vi "禹山电导率_获取温度和测量值.vi"(8 "error in (no error)":errorcluster caption="错误输入（无错误）", 11 "MB session in":refnum<class "MB_Master.lvclass">) -> (0 "error out":errorcluster caption="错误输出", 2 "输出值":cluster{"温度测量值":sgl, "电导率":sgl, "错误标志":u16} {"错误标志" items=["NO Error"=0, "量程切换错误标识"=255]}, 3 "MB session out":refnum<class "MB_Master.lvclass">)   [LabVIEW 2016, in "斯坦道多参数.lvlib"]
uses:
  <vilib>/Plasmionique/MB Master/MB_Master/MB_Master.lvclass
  <vilib>/Plasmionique/MB Master/MB Master.lvlib
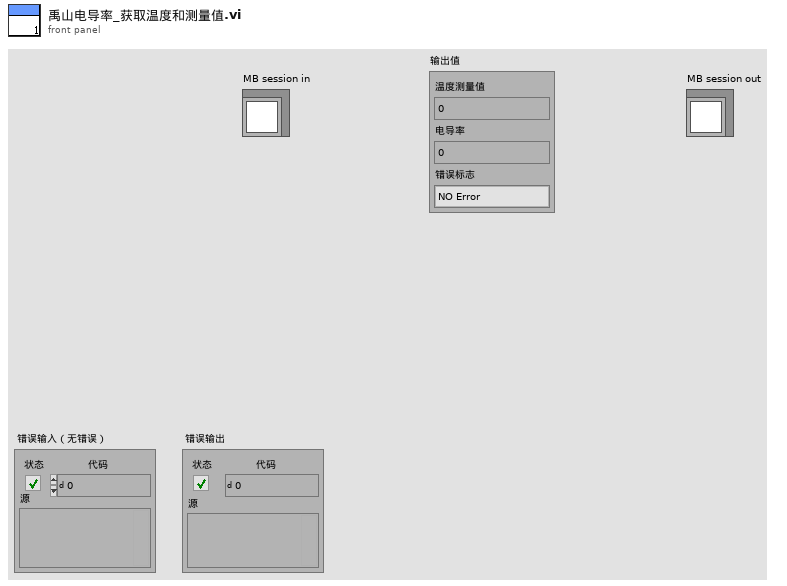
[diagram p1: front panel]
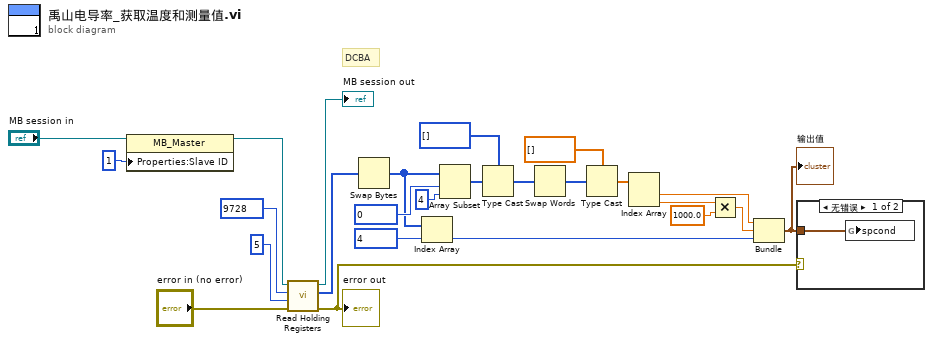
[diagram p0: block diagram]
diagram:
  # "DCBA"
  n1 = property class="MB_Master"(reference="MB session in", "Properties:Slave ID"=u16 1 ("y")) -> (reference out=w17:refnum<class "MB_Master.lvclass">)  [unwired: 1 in, 1 out]
  n2 = call <vilib>:"Read Holding Registers.vi"("error in (no error)"="error in (no error)", "quantity"=u16 5, "starting address"=u16 9728, "MB session in"=w17) -> ("error out"=w10:errorcluster, "Registers"=w15:u16[], "MB session out"=→"MB session out":refnum<class "MB_Master.lvclass">)  [unwired: 5 in]
  "error out" <- w10
  n3 = Swap Bytes(anything=w15) -> (byte swapped=w4:u16[])
  n4 = Index Array(array=w4, index=u16 4 ("starting address")) -> (element=w3:u16)
  n5 = Array Subset(array=w4, index=u16 0 ("starting address"), length=4 ("长度")) -> (w8:u16[])
  n6 = Type Cast(type=u32[] [] ("数组 2"), x=w8) -> (*(type *) &x=w21:u32[])
  n7 = Swap Words(1:w21) -> (0:w23:u32[])
  n8 = Type Cast(type=sgl[] [] ("数组 2"), x=w23) -> (*(type *) &x=w19:sgl[])
  n9 = Index Array(array=w19) -> (element #1=w14:sgl, element #2=w13:sgl)  [unwired: 2 in]
  n10 = Multiply(x=w13, y=sgl 1000.0) -> (x*y=w12:sgl)
  n11 = Bundle("数值"=w14, w12, w3) -> (w9:cluster{"数值":sgl, sgl, u16})  [unwired: 1 in]
  "输出值" <- w9
  n12 = case shown="无错误" w10 {
    tunnel: w9 -> [w26 _]
    frame No Error {
      n13 = global write "禹山过程全局变量.vi" "spcond"(w26) -> ()
    }
    frame Error {
    }
  }
